vi "Send Request Message.vi"(8 "error in (no error)":errorcluster, 10 "Message":refnum<class "Message.lvclass">, 11 "Actor API in":refnum<class "Actor API.lvclass">) -> (0 "error out":errorcluster)   [LabVIEW 2015, in "Actor API.lvclass"]
uses:
  Actor API.lvclass
  Messaging/Message/Message.lvclass
  Actor API.lvclass/Actor API.ctl
  Messaging/Messenger/Messenger.lvclass/Messenger.ctl
  Messaging/Message/Message.lvclass/Message.ctl
  Messaging/Message/get Priority.vi
  Messaging/Messenger/Messenger.lvclass
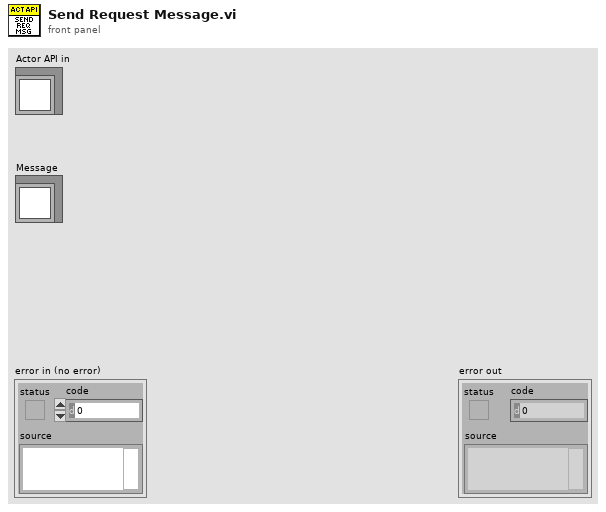
[diagram p1: front panel]
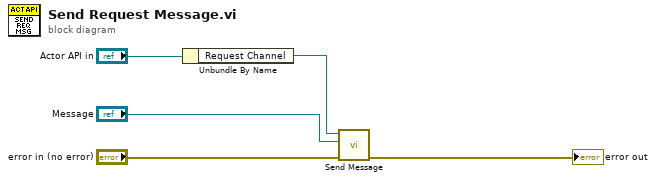
[diagram p0: block diagram]
diagram:
  n1 = Unbundle By Name("Actor API in") -> ("Request Channel"=w1:refnum<class "Messenger.lvclass">)
  n2 = call "Send Message.vi"("error in (no error)"="error in (no error)", "Message In"="Message", "Messenger in"=w1) -> ("error out"=→"error out":errorcluster)  [unwired: 8 in]
